vi "AfterPage2_UI.vi"(10 "MetaDataObj":refnum<class "MetaDataObj.lvclass">) -> ()   [LabVIEW 2021, in "Plugin_Generator.lvclass"]
uses:
  Plugin_Generator.lvclass
  <resource>/dialog/NewProjectWizard/MetaDataObj/MetaDataObj.lvclass
  Plugin_Generator.lvclass/Plugin_Generator.ctl
  <resource>/dialog/NewProjectWizard/MetaDataObj/MetaDataObj.lvclass/MetaDataObj.ctl
  <resource>/dialog/NewProjectWizard/MetaDataObj/Accessors/Read Project Name.vi
  <resource>/dialog/NewProjectWizard/MetaDataObj/Accessors/Read Project Root.vi
  <resource>/dialog/NewProjectWizard/Project Copying/NI_NPW_Project Copying.lvlib
  <vilib>/CIF Foundation/CIF Channels Core/CIFChannels/Typedef/Direction.ctl
  <vilib>/CIF Foundation/CIF Channels Core/CIFChannels/CIFChannels.lvclass
  Channels/ChannelRegistrar/typedef/Registered Channel Types.ctl
  Channels/ChannelRegistrar/ChannelRegistrar.lvlib
  Channels/ChannelRegistrar/typedef/Channel Definition for Scripting.ctl
panel:
  out "Channels to Create":T1[](array[typedef])
  out "Project Root":path
  out "Project Name":string
  out "Payload Name":string
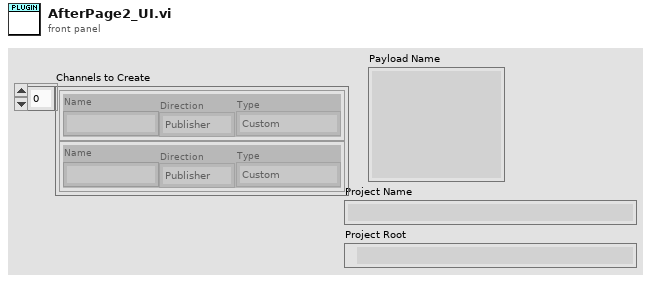
[diagram p1: front panel]
types:
  T1 = typedef "ChannelRegistrar.lvlib/Channel Definition for Scripting.ctl" = cluster{"Name":string, "Direction":T2, "Type":T3}
  T2 = typedef "CIFChannels.lvclass/Direction.ctl" = enum16{"Publisher", "Subscriber"}
  T3 = typedef "ChannelRegistrar.lvlib/Registered Channel Types.ctl" = enum16{"Custom", "Double_Tag", "I64_Tag", "U64_Tag", "U8_FIFO", "CAN_FIFO", "L2Enet_FIFO", "DAQ_FIFO", "Universal_FIFO", "String_Tag"}
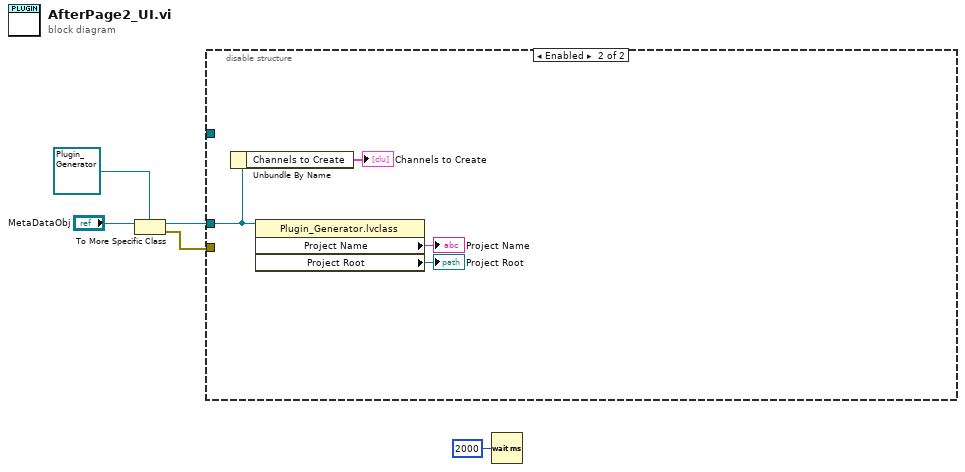
[diagram p0: block diagram]
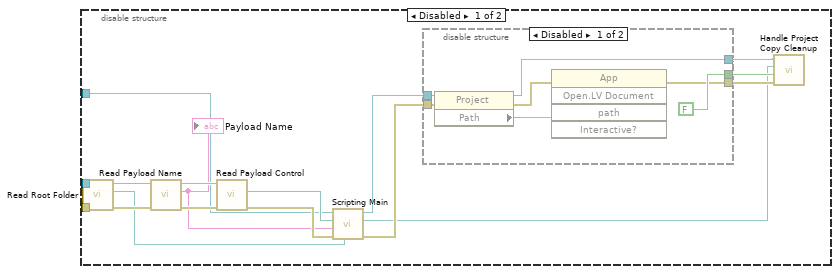
[diagram p2: hidden frame]
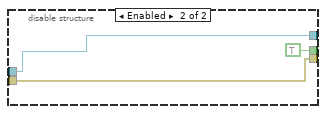
[diagram p3: hidden frame]
diagram:
  n1 = To More Specific Class(target class=refnum<class "Plugin_Generator.lvclass"> refnum ("Plugin_Generator.lvclass"), reference="MetaDataObj") -> (specific class reference=w3:refnum<class "Plugin_Generator.lvclass">, error out=w2:errorcluster)  [unwired: 1 in]
  n2 = disable-structure shown="Enabled" {
    disable-tunnel: w2 -> [w18 _]
    disable-tunnel: w3 -> [w17 w34]
    disable-tunnel: _ -> [w10 _]
    frame Disabled {
      n3 = call "Read Root Folder.vi"("error in"=w18, "NIADASReplayHIL_Channel_MetaDataObj in"=w17) -> ("error out"=w15:errorcluster, "Root Folder"=w12:path, "NIADASReplayHIL_Channel_MetaDataObj out"=w16:refnum<class "NIADASReplayHIL_Channel_MetaDataObj.lvclass">)  [unwired: 7 in]
      n4 = call "Read Payload Name.vi"("error in"=w15, "NIADASReplayHIL_Channel_MetaDataObj in"=w16) -> ("error out"=w21:errorcluster, "Payload Name"=w13:string, "NIADASReplayHIL_Channel_MetaDataObj out"=w22:refnum<class "NIADASReplayHIL_Channel_MetaDataObj.lvclass">)  [unwired: 7 in]
      "Payload Name" <- w13
      n5 = call "Read Payload Control.vi"("error in"=w21, "NIADASReplayHIL_Channel_MetaDataObj in"=w22) -> ("error out"=w14:errorcluster, "Payload Control"=w11:path)  [unwired: 7 in, 1 out]
      n6 = call "Scripting Main.vi"("Root Folder"=w12, "error in"=w14, "Payload Name (\"_Payload\" will be added by default)"=w13, "Payload Control"=w11, "User Project"=w10) -> ("error out"=w19:errorcluster, "Payload Folder Path"=w6:path, "User Project out"=w20:refnum<vi>)  [unwired: 4 in]
      n7 = disable-structure shown="Disabled" {
        disable-tunnel: w20 -> [w27 w30]
        disable-tunnel: w19 -> [w26 w32]
        disable-tunnel: [FALSE ("More Scripting?") TRUE ("More Scripting?")] -> w9
        disable-tunnel: [w24 w32] -> w8
        disable-tunnel: [w23 w30] -> w7
        frame Disabled {
          n8 = property class="Project"(reference=w27, error in=w26) -> (reference out=w23:refnum<vi>, error out=w28:errorcluster, "Path"=w29:path)
          n9 = invoke class="App" method="Open.LV Document"(error in=w28, "path"=w29) -> (error out=w24:errorcluster)  [unwired: 3 in, 4 out]
        }
        frame Enabled {
        }
      }
      n10 = call <resource>:"Handle Project Copy Cleanup.vi"("error in (no error)"=w8, "More Scripting?"=w9, "Target Path"=w6, "Project in"=w7) -> ()  [unwired: 8 in]
    }
    frame Enabled {
      n11 = Unbundle By Name(w34) -> ("Channels to Create"=→"Channels to Create":T1[])
      n12 = property class="Plugin_Generator.lvclass"(reference=w34) -> ("Project Name"=→"Project Name":string, "Project Root"=→"Project Root":path)  [unwired: 1 in, 2 out]
    }
  }
  n13 = Wait (ms)(milliseconds to wait=u32 2000) -> ()  [unwired: 1 out]
